vi "writeToXML.vi"(8 "error in (no error)":errorcluster, 10 "ClassLabel":string, 11 "Guide in":refnum<class "Guide.lvclass">) -> (0 "error out":errorcluster, 2 "XML out":string, 3 "Guide out":refnum<class "Guide.lvclass">)   [LabVIEW 2014, in "TCSDataDefinitions.lvlib" / "TCSCommand.lvlib" / "GuiderCommands.lvlib" / "Guide.lvclass"]
uses:
  Guide.lvclass
  Guide.lvclass/Guide.ctl
  GuiderCommands.lvclass
  <userlib>/Common/XML/XMLGenerator/XMLGenerator.lvclass
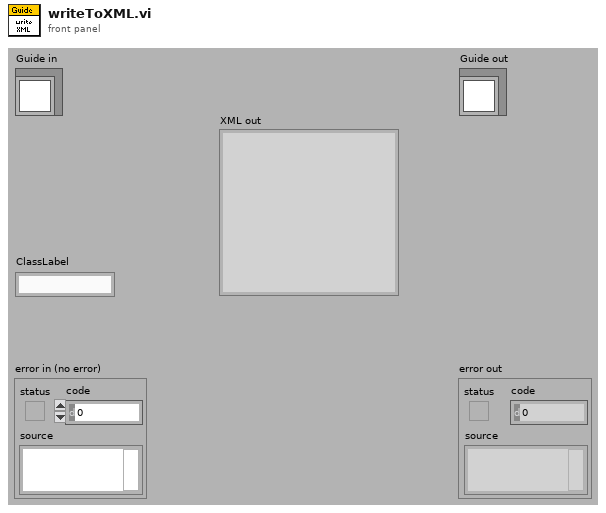
[diagram p1: front panel]
types:
  T1 = typedef "TCSDataDefinitions.lvlib/TCSCommand.lvlib/GuideStateTypes.ctl" = enum16{"On", "Off"}
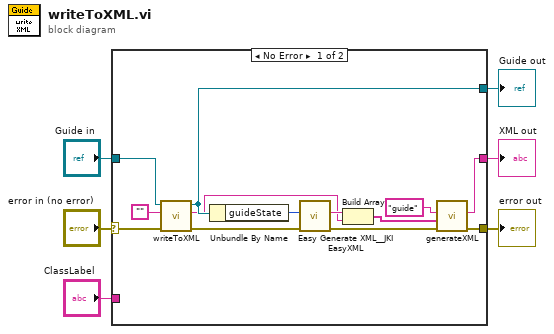
[diagram p0: block diagram]
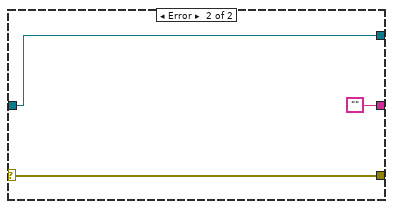
[diagram p2: hidden frame]
diagram:
  n1 = case shown="No Error" "error in (no error)" {
    selector: "error in (no error)" -> [w13 w22]
    tunnel: [w10 w22] -> w5
    tunnel: [w18 w21] -> w3
    tunnel: "Guide in" -> [w19 w21]
    tunnel: "ClassLabel" -> [_ _]
    tunnel: [w9 ""] -> w1
    frame No Error {
      n2 = call-parent "writeToXML.vi"("error in (no error)"=w13, "ClassLabel"="", "GuiderCommands in"=w19) -> ("error out"=w12:errorcluster, "XML out"=w15:string, "GuiderCommands out"=w18:refnum<class "Guide.lvclass">)  [unwired: 6 in]
      n3 = Unbundle By Name(w18) -> ("guideState"=w17:T1)
      n4 = call <vilib>:"Easy Generate XML__JKI EasyXML.vi"("error in (no error)"=w12, "LabVIEW Data"=w17) -> ("error out"=w11:errorcluster, "XML String"=w16:string)  [unwired: 8 in]
      n5 = Build Array(w16, w15) -> (w8:string[])
      n6 = call <userlib>:"generateXML.vi"("error in"=w11, "childrenXML"=w8, "elementName"="guide" ("Class Label")) -> ("error out"=w10:errorcluster, "XML out"=w9:string)  [unwired: 6 in, 1 out]
    }
    frame Error {
    }
  }
  "error out" <- w5
  "Guide out" <- w3
  "XML out" <- w1
